vi "Configure Common.vi"(8 "error in (no error)":errorcluster, 10 "Common Configuration":T1={"Tuner Mode"=1, "Calibration ID"=1, "DUT to Tuner S-parameters"=[{"S11"=0.0+0.0i, "S21"=1.0+0.0i, "S12"=1.0+0.0i, "S22"=0.0+0.0i}], "Load Termination"=[0.0+0.0i]} {"Tuner Mode" items=["Source", "Load"]}, 11 "iTuner reference in":refnum<k7>) -> (0 "error out":errorcluster, 2 "Primary Frequency (GHz)":dbl, 3 "iTuner reference out":refnum<k7>)   [LabVIEW 2016, in "FocusTuner.lvlib"]
doc: "Configures common settings for load pull using the Focus tuner."
uses:
  FocusTuner.lvlib
  Typedefs/Common Configuration.ctl
  Typedefs/S Parameter.ctl
  <instrlib>/Focus iTuner Series/Focus iTuner Series.lvlib
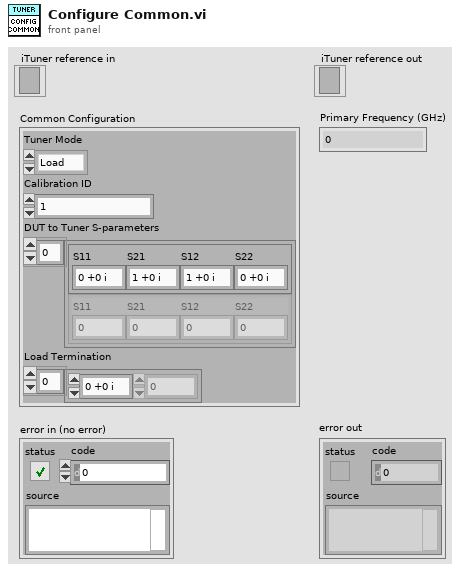
[diagram p1: front panel]
types:
  T1 = typedef "FocusTuner.lvlib/Common Configuration.ctl" = cluster{"Tuner Mode":u16, "Calibration ID":i32, "DUT to Tuner S-parameters":T2[], "Load Termination":cdb[]}
  T2 = typedef "FocusTuner.lvlib/S Parameter.ctl" = cluster{"S11":cdb, "S21":cdb, "S12":cdb, "S22":cdb}
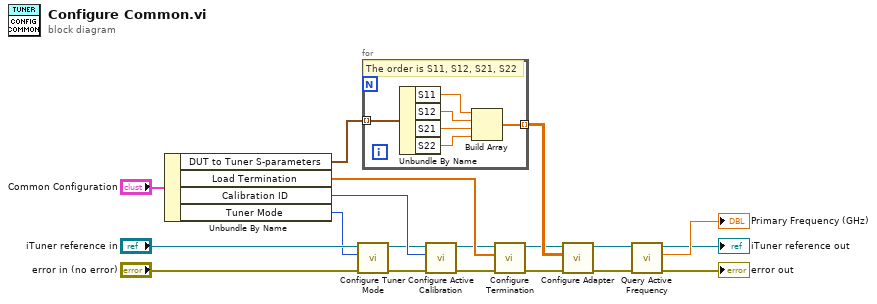
[diagram p0: block diagram]
diagram:
  n1 = Unbundle By Name("Common Configuration") -> ("DUT to Tuner S-parameters"=w12:T2[], "Load Termination"=w13:cdb[], "Calibration ID"=w14:i32, "Tuner Mode"=w15:u16)
  n2 = call <instrlib>:"Configure Tuner Mode.vi"("error in (no error)"="error in (no error)", "Tuner Mode (0: Source)"=w15, "iTuner reference in"="iTuner reference in") -> ("error out"=w4:errorcluster, "iTuner reference out"=w8:refnum<k7>)  [unwired: 7 in]
  n3 = for {
    tunnel: w12 -> [w25] mode=indexing
    tunnel: [w20] -> w11 mode=indexing
    # "The order is S11, S12, S21, S22"
    n4 = Unbundle By Name(w25) -> ("S11"=w24:cdb, "S12"=w23:cdb, "S21"=w22:cdb, "S22"=w21:cdb)
    n5 = Build Array(w24, w23, w22, w21) -> (w20:cdb[])
  }
  n6 = call <instrlib>:"Configure Active Calibration.vi"("error in (no error)"=w4, "Calibration ID (0)"=w14, "iTuner reference in"=w8) -> ("error out"=w3:errorcluster, "iTuner reference out"=w7:refnum<k7>)  [unwired: 7 in]
  n7 = call <instrlib>:"Configure Termination.vi"("error in (no error)"=w3, "Termination"=w13, "iTuner reference in"=w7) -> ("error out"=w2:errorcluster, "iTuner reference out"=w6:refnum<k7>)  [unwired: 7 in]
  n8 = call <instrlib>:"Configure Adapter.vi"("error in (no error)"=w2, "S-parameters"=w11, "iTuner reference in"=w6) -> ("error out"=w1:errorcluster, "iTuner reference out"=w5:refnum<k7>)  [unwired: 7 in]
  n9 = call <instrlib>:"Query Active Frequency.vi"("error in (no error)"=w1, "iTuner reference in"=w5) -> ("error out"=→"error out":errorcluster, "Primary Frequency (GHz)"=→"Primary Frequency (GHz)":dbl, "iTuner reference out"=→"iTuner reference out":refnum<k7>)  [unwired: 6 in, 1 out]
